vi "Log.vi"(10 "Log Packet":T1, 11 "Network Sink in":refnum<class "Network Sink.lvclass">) -> (0 "error out":errorcluster, 3 "Network Sink out":refnum<class "Network Sink.lvclass">)   [LabVIEW 2017, in "Network Sink.lvlib" / "Network Sink.lvclass"]
uses:
  <vilib>/gpm_packages/@cs/event-logger/Source/Network Sink/Network Sink/Network Sink.lvclass
  <vilib>/gpm_packages/@cs/event-logger/Source/Composed Log/Types/Log Packet.ctl
  <vilib>/gpm_packages/@cs/event-logger/Source/Composed Log/Types/Log Level.ctl
  <vilib>/gpm_packages/@cs/event-logger/Source/Network Sink/Network Sink/Network Sink.lvclass/Network Sink.ctl
  <vilib>/gpm_packages/@cs/event-logger/Source/Composed Log/Composed Log.lvlib
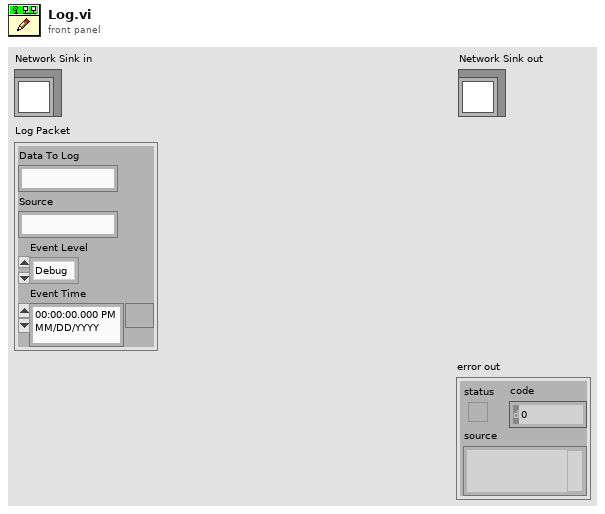
[diagram p1: front panel]
types:
  T1 = typedef "Composed Log.lvlib/Log Packet.ctl" = cluster{"Data To Log":string, "Source":string, "Event Level":T2, "Event Time":timestamp}
  T2 = typedef "Composed Log.lvlib/Log Level.ctl" = enum16{"Debug", "Info", "Warning", "Error", "Critical"}
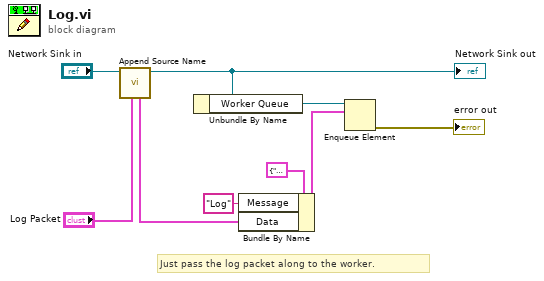
[diagram p0: block diagram]
diagram:
  # "Just pass the log packet along to the worker."
  n1 = call <vilib>:"Append Source Name.vi"("Log Packet"="Log Packet", "Network Sink in"="Network Sink in") -> ("Network Sink out"=w3:refnum<class "Network Sink.lvclass">, "Log Packet  Out"=w1:T1)  [unwired: 8 in]
  "Network Sink out" <- w3
  n2 = Unbundle By Name(w3) -> ("Worker Queue"=w9:refnum<queue>)
  n3 = Bundle By Name(cluster=cluster{"Message":string, "Data":variant} {"Message"="", "Data"=variant} ("element"), "Message"="Log", "Data"=w1) -> (w7:cluster{"Message":string, "Data":variant})
  n4 = Enqueue Element(queue=w9, element=w7) -> (error out=→"error out":errorcluster)  [unwired: 2 in, 2 out]
